vi "PAN_GetCmdQ.vi"() -> (1 "cmd struct":T1, 2 "cmdQ":refnum<queue>)   [LabVIEW 2016]
uses:
  private/vis/PAN_cmdStruct.ctl
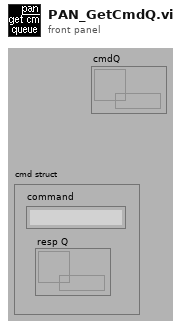
[diagram p1: front panel]
types:
  T1 = typedef "PAN_cmdStruct.ctl" = cluster{"command":string, "resp Q":refnum<queue>}
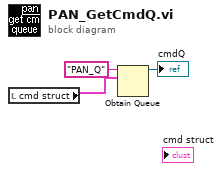
[diagram p0: block diagram]
diagram:
  n1 = local read "cmd struct"() -> (w1:T1)
  n2 = Obtain Queue(name (unnamed)="PAN_Q", element data type=w1) -> (queue out=→"cmdQ":refnum<queue>)  [unwired: 3 in, 2 out]
